vi "Configure Channel.vi"(4 "Impedance (1E+6 Ohms)":i32(ring)=1000000 items=["50"=50, "75"=75, "1E+6"=1000000], 6 "Attenuation (1:1)":u16(ring)=1 items=["1"=1, "10"=10], 7 "Enable Filter (F:Disable)":bool, 8 "error in (no error)":errorcluster, 9 "Coupling (0:AC)":i32(ring) items=["AC", "DC"], 10 "Channel (1:Channel 1)":i32(ring)=1 items=["Channel 1"=1, "Channel 2"=2], 11 "VISA resource name":refnum<visa-resource-name>) -> (0 "error out":errorcluster, 3 "VISA resource name out":refnum<visa-resource-name>)   [LabVIEW 2015, in "Template - Counter.lvlib"]
doc: "Configures the characteristics of the channel to which an input is connected."
uses:
  <instrlib>/_Template - Counter/Template - Counter.lvlib
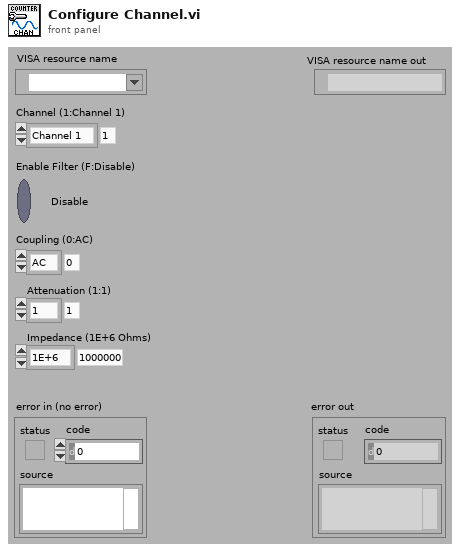
[diagram p1: front panel]
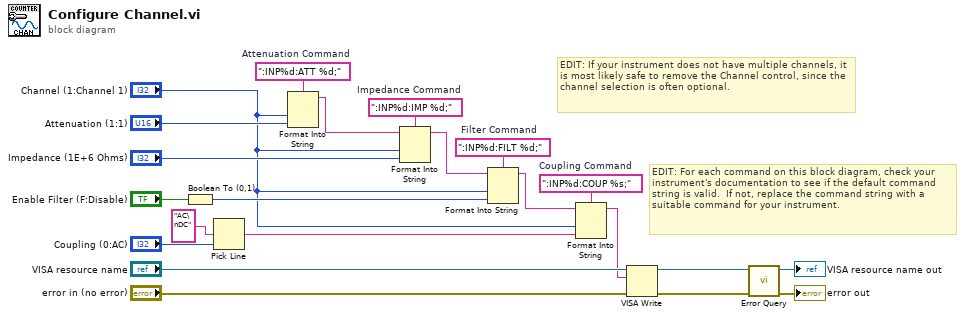
[diagram p0: block diagram]
diagram:
  w10 = ":INP%d:COUP %s;"  # Coupling Command
  w11 = ":INP%d:FILT %d;"  # Filter Command
  w12 = ":INP%d:IMP %d;"  # Impedance Command
  w13 = ":INP%d:ATT %d;"  # Attenuation Command
  # "EDIT: If your instrument does not have multiple channels, it is most likely safe to remove the Channel control, since the channel selection is often optional."
  # "EDIT: For each command on this block diagram, check your instrument's documentation to see if the default command string is valid.  If not, replace the command string with a suitable command for your instrument."
  n1 = Boolean To (0,1)(Boolean="Enable Filter (F:Disable)") -> (0, 1=w7:i16)
  n2 = Pick Line(multi-line string="AC\nDC" ("format string"), line index="Coupling (0:AC)") -> (output string=w8:string)  [unwired: 1 in]
  n3 = Format Into String(format string=w13, "Channel (1:Channel 1)", "Attenuation (1:1)") -> (resulting string=w2:string)  [unwired: 2 in, 1 out]
  n4 = Format Into String(format string=w12, initial string=w2, "Channel (1:Channel 1)", "Impedance (1E+6 Ohms)") -> (resulting string=w3:string)  [unwired: 1 in, 1 out]
  n5 = Format Into String(format string=w11, initial string=w3, "Channel (1:Channel 1)", w7) -> (resulting string=w4:string)  [unwired: 1 in, 1 out]
  n6 = Format Into String(format string=w10, initial string=w4, "Channel (1:Channel 1)", w8) -> (resulting string=w5:string)  [unwired: 1 in, 1 out]
  n7 = VISA Write(VISA resource name="VISA resource name", write buffer=w5, error in (no error)="error in (no error)") -> (VISA resource name out=w19:refnum<visa-resource-name>, error out=w17:errorcluster)  [unwired: 1 out]
  n8 = call <instrlib>:"Error Query.vi"("error in (no error)"=w17, "VISA resource name"=w19) -> ("error out"=→"error out":errorcluster, "VISA resource name out"=→"VISA resource name out":refnum<visa-resource-name>)  [unwired: 6 in, 2 out]
